vi "Format Rate.vi"(10 "Rate":dbl) -> (2 "String":string)   [LabVIEW 2017, in "Cobertura.lvlib"]
doc: "Returns a numerical string representation of the provided rate."
uses:
  Cobertura.lvlib
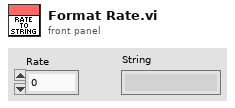
[diagram p1: front panel]
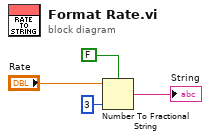
[diagram p0: block diagram]
diagram:
  n1 = Number To Fractional String(use system decimal point (T)=FALSE, number="Rate", precision (6)=i16 3) -> (F-format string=→"String":string)  [unwired: 1 in]
